vi "p41 bordes mascara.vi"() -> ()   [LabVIEW 2017]
uses:
  <vilib>/Analysis/Matrix/Datatypes/RealMatrix.ctl
  <vilib>/Analysis/Matrix/Numeric/Conversions/Array To Matrix - RA2.vi
  <vilib>/Analysis/Matrix/Numeric/Conversions/Matrix To Array - RM.vi
  <vilib>/Analysis/Matrix/NI_Matrix.lvlib
panel:
  out "output matrix":T1
  out "new picture 3":picture
  out "new picture 2":picture
  in  "path to JPEG file":path
  in  "Slide":dbl(slide) scale=0.0..255.0
  in  "path to BMP file":path
  out "new picture":picture
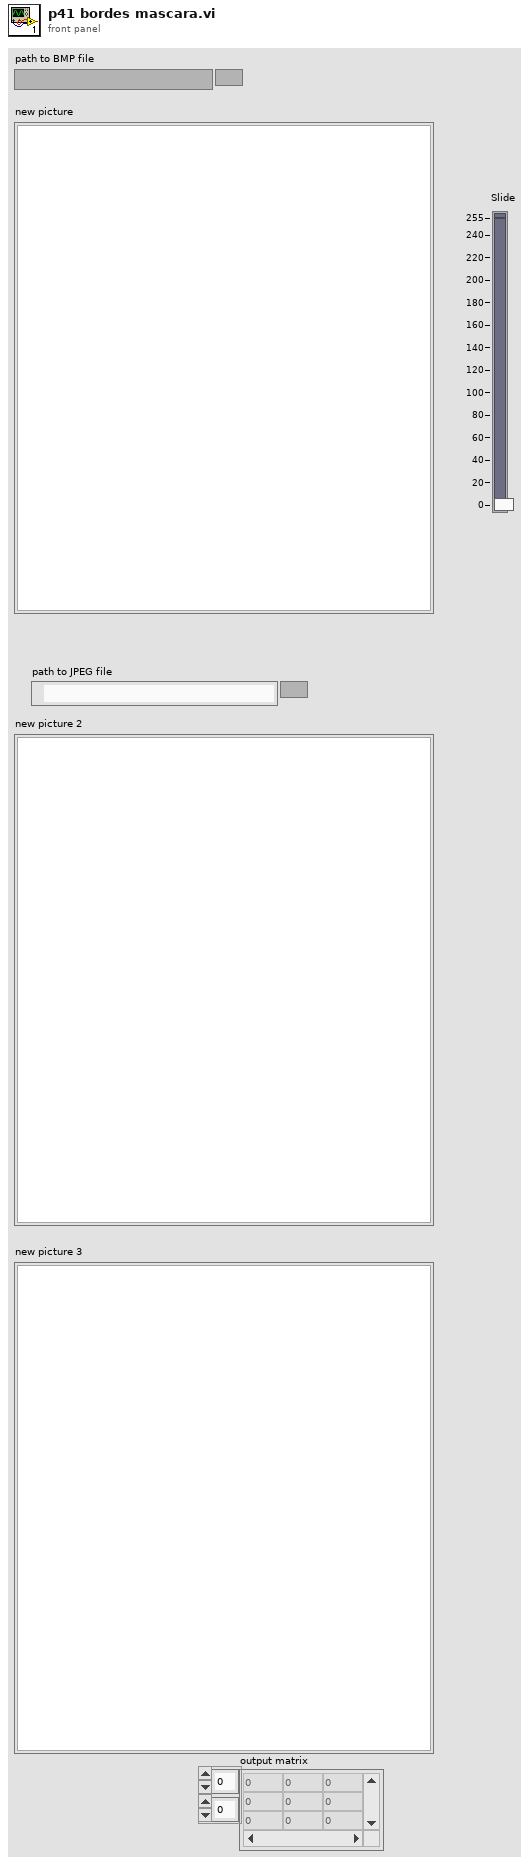
[diagram p1: front panel]
types:
  T1 = typedef "NI_Matrix.lvlib/RealMatrix.ctl" = dbl[][]
  T2 = typedef "imagedata.ctl" = cluster{"image type":i32, "image depth":i32, "image":u8[], "mask":u8[], "colors":u32[], "Rectangle":cluster{"left":i16, "top":i16, "right":i16, "bottom":i16}}
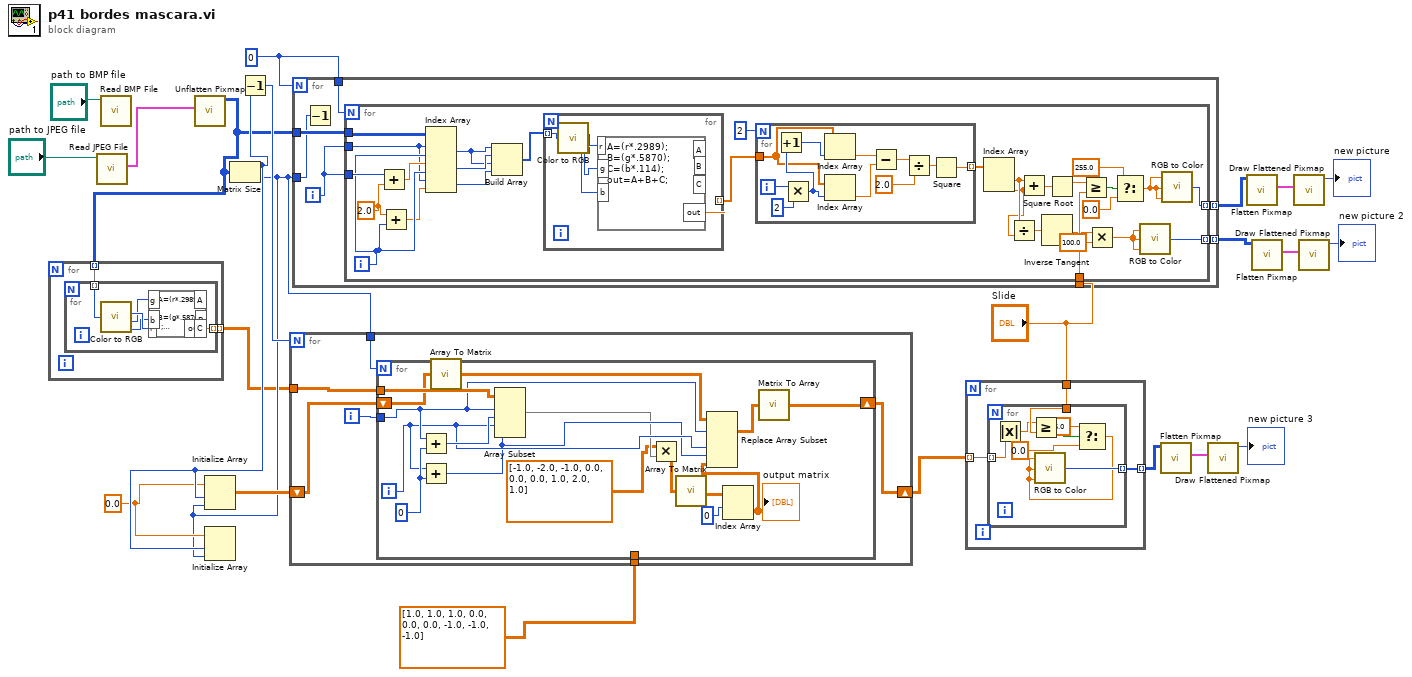
[diagram p0: block diagram]
diagram:
  w6 = 0
  w12 = 0.0 ("element")
  n1 = call <vilib>:"Read JPEG File.vi"("path to JPEG file"="path to JPEG file") -> ("image data"=w19:T2)  [unwired: 8 in, 2 out]
  n2 = call <vilib>:"Read BMP File.vi"("path to BMP file"="path to BMP file") -> ()  [unwired: 8 in, 3 out]
  n3 = call <vilib>:"Unflatten Pixmap.vi"("image data"=w19) -> ("24-bit pixmap"=w2:u32[][])  [unwired: 4 in, 6 out]
  n4 = for {
    tunnel: w2 -> [w25] mode=indexing
    tunnel: [w24] -> w1 mode=indexing
    n5 = for {
      tunnel: w25 -> [w30] mode=indexing
      tunnel: [w26] -> w24 mode=indexing
      n6 = call <vilib>:"Color to RGB.vi"("Color"=w30) -> ("R"=w29:u8, "G"=w28:u8, "B"=w27:u8)  [unwired: 1 out]
      n7 = formula code="A=(r*.2989);\nB=(g*.5870);\nC=(b*.114);\nout=A+B+C;"("r"=w29, "g"=w28, "b"=w27) -> ("out"=w26:dbl)  [unwired: 3 out]
    }
  }
  n8 = Matrix Size(0:w2) -> (1:w13:i32, 2:w5:i32)
  n9 = Initialize Array(w12, w13, w5) -> (w8:dbl[][])
  n10 = Initialize Array(w12, w13, w5) -> ()  [unwired: 1 out]
  n11 = Decrement(x=w13) -> (x-1=w14:i32)
  n12 = for {
    N: w14 -> [_]
    tunnel: w1 -> [w36]
    shift-right: [w33] -> w7
    shift-left: w8 -> [w34]
    tunnel: w5 -> [w32]
    tunnel: dbl[][] [[1.0, 1.0, 1.0], [0.0, 0.0, 0.0], [-1.0, -1.0, -1.0]] -> [w31]
    i -> [w35]
    n13 = for {
      N: w32 -> [_]
      tunnel: w36 -> [w52]
      tunnel: w35 -> [w41]
      shift-right: [w48] -> w33
      shift-left: w34 -> [w51]
      tunnel: w31 -> [_]
      i -> [w40]
      w44 = 0
      n14 = Add(x=w41, y=w44) -> (x+y=w45:i32)
      n15 = Add(x=w40, y=w44) -> (x+y=w39:i32)
      n16 = call-poly <vilib>:"Array To Matrix.vi"("Real 2D Array"=w51) -> ("Real Matrix"=w50:T1)
      n17 = Array Subset(array=w52, index (row)=w41, length (row)=w45, index (col)=w40, length (col)=w39) -> (w38:dbl[][])
      n18 = Multiply ("Multiply.vi")(x=dbl[][] [[-1.0, -2.0, -1.0], [0.0, 0.0, 0.0], [1.0, 2.0, 1.0]], y=w38) -> (x*y=w47:dbl[][])
      n19 = call-poly <vilib>:"Array To Matrix.vi"("Real 2D Array"=w47) -> ("Real Matrix"=w46:T1)
      n20 = Index Array(array=w46, index (row)=0 ("index (col)")) -> (element=w42:T1)  [unwired: 1 in]
      "output matrix" <- w42
      n21 = Replace Array Subset(array=w50, new element=w42, index (dim 0)=w41, index (dim 2)=w40, index (dim 3)=w39) -> (w49:T1)  [unwired: 1 in]
      n22 = call-poly <vilib>:"Matrix To Array.vi"("Real Matrix"=w49) -> ("Real 2D Array"=w48:dbl[][])
    }
  }
  n23 = for {
    N: w6 -> [_]
    tunnel: w2 -> [w59]
    tunnel: w5 -> [w58]
    tunnel: [w56] -> w23 mode=indexing
    tunnel: "Slide" -> [w55]
    tunnel: [w54] -> w15 mode=indexing
    tunnel: w6 -> [w53]
    i -> [w57]
    n24 = Decrement(x=w58) -> ()  [unwired: 1 out]
    n25 = for {
      N: w53 -> [_]
      tunnel: w59 -> [w88]
      tunnel: w57 -> [w74]
      tunnel: w57 -> [w87]
      tunnel: [w77] -> w56 mode=indexing
      tunnel: w55 -> [w70]
      tunnel: [w66] -> w54 mode=indexing
      i -> [w82]
      w83 = 2.0 ("y")
      n26 = Add(x=w87, y=w83) -> (x+y=w86:dbl)
      n27 = Add(x=w83, y=w82) -> (x+y=w73:dbl)
      n28 = Index Array(array=w88, index (row) #1=w74, index (col) #1=w82, index (row) #2=w86, index (col) #2=w82, index (row) #3=w74, index (col) #3=w73) -> (element #1=w76:u32, element #2=w85:u32, element #3=w75:u32)
      n29 = Build Array(w76, w85, w76, w75) -> (w84:u32[])
      n30 = for {
        tunnel: w84 -> [w101] mode=indexing
        tunnel: [w100] -> w80 mode=indexing
        n31 = call <vilib>:"Color to RGB.vi"("Color"=w101) -> ("R"=w104:u8, "G"=w103:u8, "B"=w102:u8)  [unwired: 1 out]
        n32 = formula code="A=(r*.2989);\nB=(g*.5870);\nC=(b*.114);\nout=A+B+C;"("r"=w104, "g"=w103, "b"=w102) -> ("out"=w100:dbl)  [unwired: 3 out]
      }
      n33 = for {
        N: 2 -> [_]
        tunnel: w80 -> [w94]
        tunnel: [w89] -> w79 mode=indexing
        i -> [w97]
        n34 = Multiply(x=w97, y=2) -> (x*y=w95:i32)
        n35 = Increment(x=w95) -> (x+1=w98:i32)
        n36 = Index Array(array=w94, index=w98) -> (element=w99:dbl)
        n37 = Index Array(array=w94, index=w95) -> (element=w93:dbl)
        n38 = Subtract(x=w99, y=w93) -> (x-y=w92:dbl)
        n39 = Divide(x=w92, y=2.0) -> (x/y=w90:dbl)
        n40 = Square(x=w90) -> (x^2=w89:dbl)
      }
      n41 = Index Array(array=w79) -> (element #1=w61:dbl, element #2=w60:dbl)  [unwired: 2 in]
      n42 = Divide(x=w61, y=w60) -> (x/y=w67:dbl)
      n43 = Add(x=w61, y=w60) -> (x+y=w78:dbl)
      n44 = Inverse Tangent(1:w67) -> (0:w64:dbl)
      n45 = Square Root(x=w78) -> (sqrt(x)=w71:dbl)
      n46 = Greater Or Equal?(x=w71, y=w70) -> (x >= y?=w72:bool)
      n47 = Multiply(x=w64, y=100.0) -> (x*y=w62:dbl)
      n48 = Select(t=255.0, s=w72, f=0.0) -> (s? t:f=w68:dbl)
      n49 = call <vilib>:"RGB to Color.vi"("B"=w62, "G"=w62, "R"=w62) -> ("Color"=w66:u32)
      n50 = call <vilib>:"RGB to Color.vi"("B"=w68, "G"=w68, "R"=w68) -> ("Color"=w77:u32)
    }
  }
  n51 = for {
    tunnel: [w107] -> w9 mode=indexing
    tunnel: w7 -> [w106] mode=indexing
    tunnel: "Slide" -> [w105]
    n52 = for {
      tunnel: [w115] -> w107 mode=indexing
      tunnel: w106 -> [w109] mode=indexing
      tunnel: w105 -> [w113]
      n53 = Absolute Value(x=w109) -> (abs(x)=w108:dbl)
      n54 = Greater Or Equal?(x=w108, y=w113) -> (x >= y?=w114:bool)
      n55 = Select(t=255.0, s=w114, f=0.0) -> (s? t:f=w110:dbl)
      n56 = call <vilib>:"RGB to Color.vi"("B"=w110, "G"=w110, "R"=w110) -> ("Color"=w115:u32)
    }
  }
  n57 = call <vilib>:"Flatten Pixmap.vi"("24-bit pixmap"=w9) -> ("image data"=w11:T2)  [unwired: 10 in]
  n58 = call <vilib>:"Draw Flattened Pixmap.vi"("image data"=w11) -> ("new picture"=→"new picture 3":picture)  [unwired: 8 in]
  n59 = call <vilib>:"Flatten Pixmap.vi"("24-bit pixmap"=w23) -> ("image data"=w22:T2)  [unwired: 10 in]
  n60 = call <vilib>:"Flatten Pixmap.vi"("24-bit pixmap"=w15) -> ("image data"=w16:T2)  [unwired: 10 in]
  n61 = call <vilib>:"Draw Flattened Pixmap.vi"("image data"=w22) -> ("new picture"=→"new picture":picture)  [unwired: 8 in]
  n62 = call <vilib>:"Draw Flattened Pixmap.vi"("image data"=w16) -> ("new picture"=→"new picture 2":picture)  [unwired: 8 in]
